vi "Msg - Receive.vi"(5 "Preview?":bool, 7 "Timeout (ms)":i32, 11 "error in (no error)":errorcluster) -> (4 "Message":T1, 8 "timed out?":bool, 15 "error out":errorcluster)   [LabVIEW 2017, in "Template.lvlib"]
doc: "Receives Messages for this Module."
uses:
  Template.lvlib
  Controls/Message.ctl
  Controls/Module - States.ctl
  Controls/Message - Queue Manager Mode.ctl
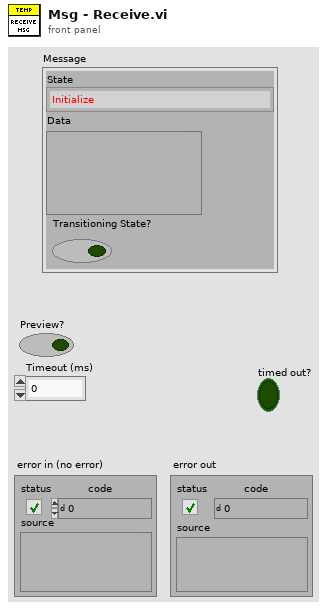
[diagram p1: front panel]
types:
  T1 = typedef "Template.lvlib/Message.ctl" = cluster{"State":T2, "Data":variant, "Transitioning State?":bool}
  T2 = typedef "Template.lvlib/Module - States.ctl" = enum16{"Initialize", "Event ", "Send data", "FP Element: Update", "FP Element: Disable/Enable", "Timer: Setup", "Terminate", "---------------Template---------------"}
  T3 = typedef "Template.lvlib/Message - Queue Manager Mode.ctl" = enum16{"Create", "Get", "Destroy"}
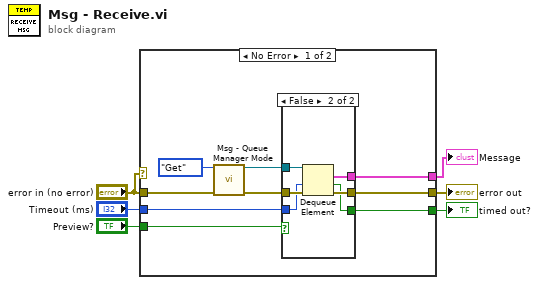
[diagram p0: block diagram]
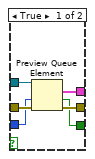
[diagram p2: hidden frame]
diagram:
  n1 = case shown="No Error" "error in (no error)" {
    tunnel: [w13 _] -> w4
    tunnel: [w11 w28] -> w6
    tunnel: "error in (no error)" -> [w12 w28]
    tunnel: "Preview?" -> [w9 _]
    tunnel: "Timeout (ms)" -> [w8 _]
    tunnel: [w7 _] -> w1
    frame No Error {
      n2 = call "Msg - Queue Manager Mode.vi"("Mode"=Message_-_Queue_Manager_Mode."Get", "error in (no error)"=w12) -> (">>ThisModule"=w10:refnum<queue>, "error out"=w14:errorcluster)  [unwired: 11 in, 1 out]
      n3 = case shown="False" w9 {
        tunnel: w14 -> [w21 w27]
        tunnel: [w20 w26] -> w13
        tunnel: [w19 w25] -> w11
        tunnel: w10 -> [w18 w24]
        tunnel: w8 -> [w17 w23]
        tunnel: [w16 w22] -> w7
        frame True {
          n4 = Preview Queue Element(queue=w18, timeout in ms (-1)=w17, error in (no error)=w21) -> (element=w20:T1, timed out?=w16:bool, error out=w19:errorcluster)  [unwired: 1 out]
        }
        frame False {
          n5 = Dequeue Element(queue=w24, timeout in ms (-1)=w23, error in (no error)=w27) -> (element=w26:T1, timed out?=w22:bool, error out=w25:errorcluster)  [unwired: 1 out]
        }
      }
    }
    frame Error {
    }
  }
  "error out" <- w6
  "Message" <- w4
  "timed out?" <- w1
